vi "Disconnect PV.vi"(8 "error in (no error)":errorcluster, 10 "PV URL":string, 11 "CS++SVMonitor in":refnum<class "CS++SVMonitor.lvclass">) -> (0 "error out":errorcluster, 3 "CS++SVMonitor out":refnum<class "CS++SVMonitor.lvclass">)   [LabVIEW 2013, in "CS++SVMonitor.lvlib" / "CS++SVMonitor.lvclass"]
doc: "Close connection to process variable."
uses:
  CS++SVMonitor.lvclass
  CS++PVMonitor/CS++PVMonitor.lvclass/CS++PVMonitor.ctl
  CS++SVMonitor.lvclass/CS++SVMonitor.ctl
  CS++PVMonitor/CS++PVMonitor.lvclass
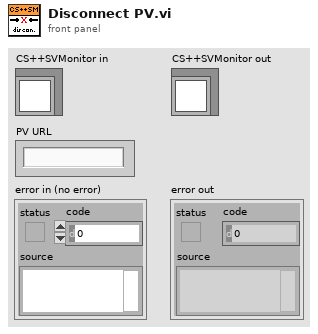
[diagram p1: front panel]
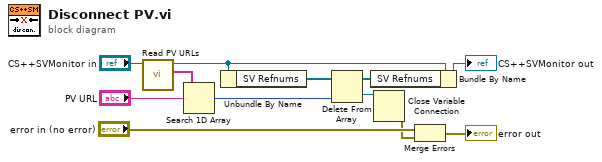
[diagram p0: block diagram]
diagram:
  n1 = call "Read PV URLs.vi"("CS++PVMonitor in"="CS++SVMonitor in") -> ("PV URLs"=w11:string[], "CS++PVMonitor out"=w7:refnum<class "CS++SVMonitor.lvclass">)  [unwired: 8 in, 1 out]
  n2 = Search 1D Array(1D array=w11, element="PV URL") -> (index of element=w8:i32)  [unwired: 1 in]
  n3 = Unbundle By Name(w7) -> ("SV Refnums"=w9:refnum<k21>[])
  n4 = Delete From Array(array=w9, index=w8) -> (deleted portion=w4:refnum<k21>, array with subset deleted=w5:refnum<k21>[])  [unwired: 1 in]
  n5 = Bundle By Name(cluster=w7, "SV Refnums"=w5) -> (→"CS++SVMonitor out":refnum<class "CS++SVMonitor.lvclass">)
  n6 = Close Variable Connection(11:w4) -> (0:w2:errorcluster)  [unwired: 1 in]
  n7 = Merge Errors("error in (no error)", w2) -> (→"error out":errorcluster)
